vi "실습 6-1 이벤트 구조 사용.vi"() -> ()   [LabVIEW 2014]
uses:
  <vilib>/Analysis/NI_AALBase.lvlib
panel:
  out "웨이브폼 그래프":dbl[](graph)
  in  "정지":bool
  in  "삼각파형":bool
  in  "사인파형":bool
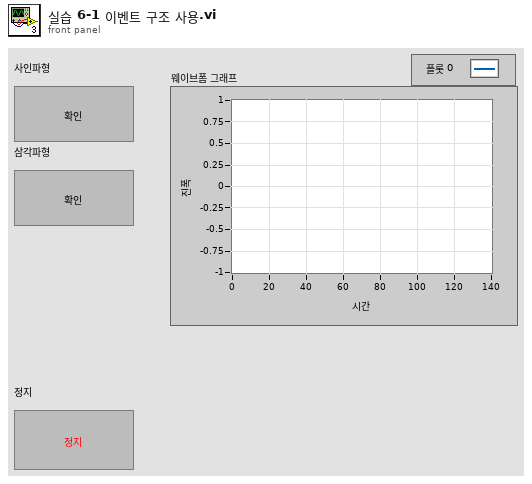
[diagram p1: front panel]
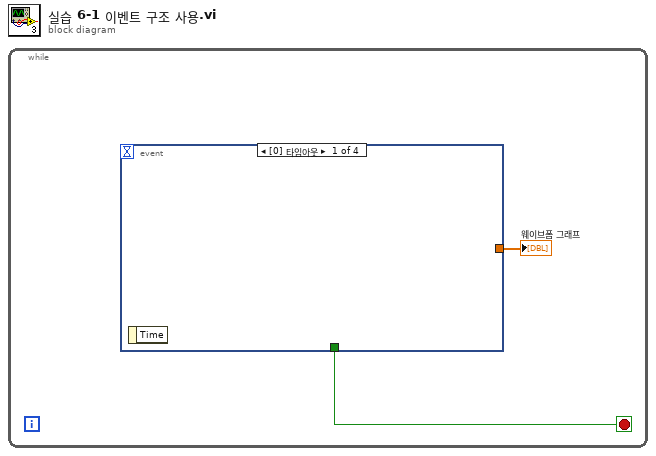
[diagram p0: block diagram]
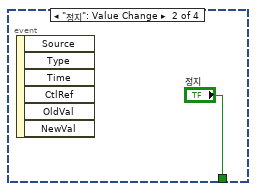
[diagram p2: hidden frame]
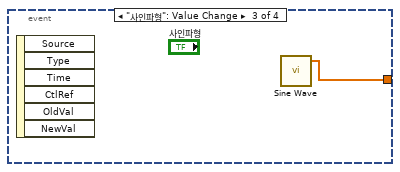
[diagram p3: hidden frame]
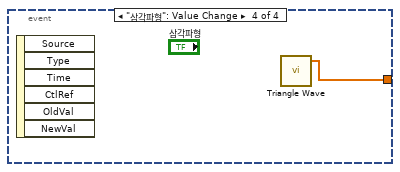
[diagram p4: hidden frame]
diagram:
  n1 = while {
    stop <- w2 stop-if-true
    n2 = event shown="[0] 타임아웃" {
      selector: _ -> [_ _ _ _]
      dyn-events: _ -> [_ _ _ _]
      timeout: _ -> [_ _ _ _]
      tunnel: [_ "정지" _ _] -> w2
      tunnel: [_ _ w4 w5] -> w1
      event Timeout {
        n3 = event-data() -> ()  [unwired: 1 in, 1 out]
      }
      event "정지": Value Change {
        n4 = event-data() -> ()  [unwired: 1 in, 6 out]
      }
      event "사인파형": Value Change {
        n5 = event-data() -> ()  [unwired: 1 in, 6 out]
        n6 = call <vilib>:"Sine Wave.vi"() -> ("sine wave"=w4:dbl[])  [unwired: 5 in, 2 out]
      }
      event "삼각파형": Value Change {
        n7 = event-data() -> ()  [unwired: 1 in, 6 out]
        n8 = call <vilib>:"Triangle Wave.vi"() -> ("triangle wave"=w5:dbl[])  [unwired: 5 in, 2 out]
      }
    }
    "웨이브폼 그래프" <- w1
  }
